vi "fl28x Initialize.vi"(8 "error in (no error)":errorcluster, 10 "ID Query (T: Check)":bool=TRUE, 11 "VISA resource name":refnum<visa-resource-name>) -> (0 "error out":errorcluster, 3 "VISA resource name out":refnum<visa-resource-name>)   [LabVIEW 2015, in "289.lvclass"]
doc: "This VI passes the addressing information in the instrument decriptor to the Instr Open VI and returns the instrument ID. You can optionally reset the instrument by setting the front panel reset control. You must run this VI before using any of the instrument driver VIs for this instrument."
uses:
  289.lvclass
panel:
  # "Check\nDon't Check"
  # "Reset\nDon't Reset"
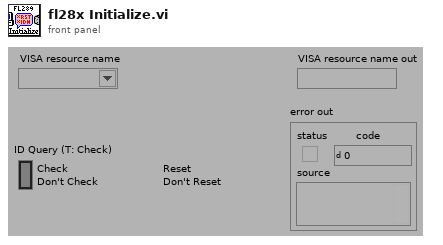
[diagram p1: front panel]
types:
  T1 = cluster{"Status":bool, "Code":i32, "Source (VI Name)":string}
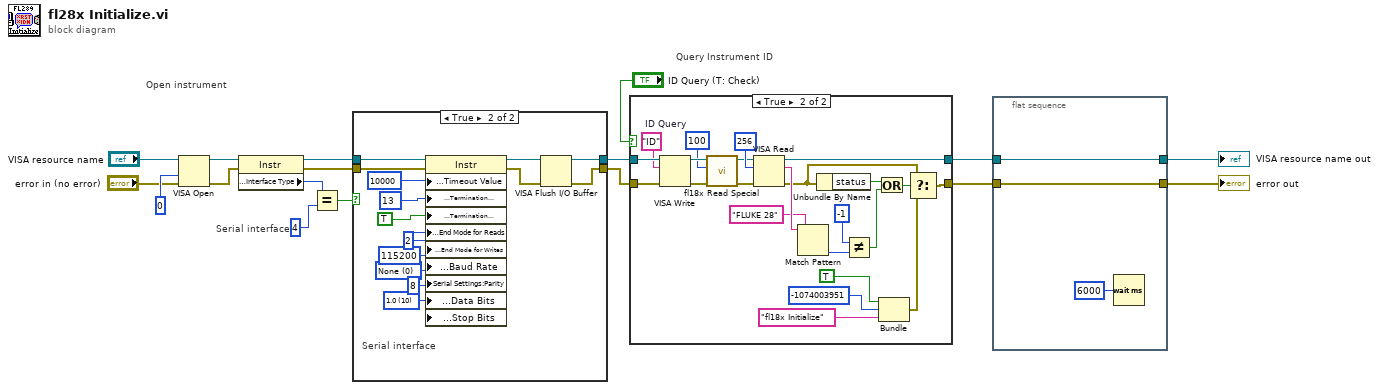
[diagram p0: block diagram]
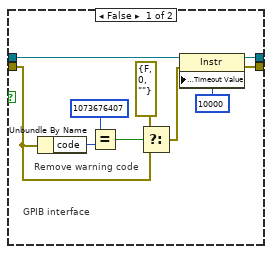
[diagram p2: hidden frame]
diagram:
  # "Serial interface"
  # "Query Instrument ID"
  # "Open instrument"
  n1 = VISA Open(access mode=u32 0, error in (no error)="error in (no error)", VISA resource name="VISA resource name") -> (VISA resource name=w15:refnum<visa-resource-name>, error out=w14:errorcluster)  [unwired: 2 in]
  n2 = property class="Instr"(reference=w15, error in=w14) -> (reference out=w10:refnum<visa-resource-name>, error out=w11:errorcluster, "Interface Information:Interface Type"=w13:u16)
  n3 = Equal?(x=w13, y=u16 4) -> (x = y?=w12:bool)
  n4 = case shown="True" w12 {
    tunnel: w11 -> [w19 w40]
    tunnel: w10 -> [w27 w41]
    tunnel: [w26 w32] -> w7
    tunnel: [w25 w34] -> w6
    frame False {
      # "Remove warning code"
      # "GPIB interface"
      n5 = Unbundle By Name(w19) -> ("code"=w20:i32)
      n6 = Equal?(x=1073676407, y=w20) -> (x = y?=w22:bool)
      n7 = Select(t=errorcluster {"status"=FALSE, "code"=0, "source"=""} ("error out"), s=w22, f=w19) -> (s? t:f=w18:errorcluster)
      n8 = property class="Instr"(reference=w27, error in=w18, "General Settings:Timeout Value"=u32 10000 ("Tmo Value")) -> (reference out=w25:refnum<visa-resource-name>, error out=w26:errorcluster)
    }
    frame True {
      w29 = u16 10 items=["1.0"=10, "1.5"=15, "2.0"=20] ("Serial Settings:Serial Stop Bits")
      w31 = u16 0 items=["None", "Odd", "Even", "Mark", "Space"] ("Serial Settings:Serial Parity")
      w36 = u16 2 ("ASRL End In")
      # "Serial interface"
      n9 = property class="Instr"(reference=w41, error in=w40, "General Settings:Timeout Value"=u32 10000, "Message Based Settings:Termination Character"=u8 13 ("TermChar"), "Message Based Settings:Termination Character Enable"=TRUE ("TermChar En"), "Serial Settings:End Mode for Reads"=w36, "Serial Settings:End Mode for Writes"=w36, "Serial Settings:Baud Rate"=u32 115200, "Serial Settings:Parity"=w31, "Serial Settings:Data Bits"=u16 8 ("Serial Settings:Serial Data Bits"), "Serial Settings:Stop Bits"=w29) -> (reference out=w35:refnum<visa-resource-name>, error out=w33:errorcluster)
      n10 = VISA Flush I/O Buffer(VISA resource name=w35, error in (no error)=w33) -> (VISA resource name out=w34:refnum<visa-resource-name>, error out=w32:errorcluster)  [unwired: 1 in]
    }
  }
  n11 = case shown="True" "ID Query (T: Check)" {
    tunnel: [w42 w66] -> w1
    tunnel: [w43 w63] -> w3
    tunnel: w6 -> [w43 w64]
    tunnel: w7 -> [w42 w65]
    frame False {
    }
    frame True {
      w52 = "ID"  # ID Query
      n12 = VISA Write(VISA resource name=w64, write buffer=w52, error in (no error)=w65) -> (VISA resource name out=w46:refnum<visa-resource-name>, error out=w47:errorcluster)  [unwired: 1 out]
      n13 = call <instrlib>:"fl18x Read Special.vi"("error in (no error)"=w47, "Byte Count (0)"=u32 100, "VISA session"=w46) -> ("error out"=w48:errorcluster, "dup VISA session"=w45:refnum<visa-resource-name>)  [unwired: 6 in, 1 out]
      n14 = VISA Read(VISA resource name=w45, byte count=u32 256, error in (no error)=w48) -> (VISA resource name out=w63:refnum<visa-resource-name>, read buffer=w60:string, error out=w59:errorcluster)  [unwired: 1 out]
      n15 = Match Pattern(string=w60, regular expression="FLUKE 28") -> (offset past match=w54:i32)  [unwired: 1 in, 3 out]
      n16 = Unbundle By Name(w59) -> ("status"=w57:bool)
      n17 = Not Equal?(x=-1, y=w54) -> (x != y?=w61:bool)
      n18 = Or(x=w57, y=w61) -> (x .or. y?=w58:bool)
      n19 = Bundle("Status"=TRUE, "Code"=-1074003951, "Source (VI Name)"="fl18x Initialize") -> (w51:T1)  [unwired: 1 in]
      n20 = Select(t=w59, s=w58, f=w51) -> (s? t:f=w66:T1)
    }
  }
  n21 = flat-sequence {
    tunnel: [w69] -> w4
    tunnel: w3 -> [w69]
    tunnel: [w68] -> w2
    tunnel: w1 -> [w68]
    frame #0 {
      n22 = Wait (ms)(milliseconds to wait=u32 6000) -> ()  [unwired: 1 out]
    }
  }
  "VISA resource name out" <- w4
  "error out" <- w2
